vi "transmit messages.vi"(5 "extended ID?":bool, 6 "Network":T1(ring), 7 "Arb ID":u32, 8 "error in":errorcluster, 9 "Number of \nData Bytes":i32, 10 "hObject In":i32, 11 "Data":u8[](array[numeric])) -> (0 "error out":errorcluster, 3 "hObject Out":i32)   [LabVIEW 2018]
uses:
  ctl networkid.ctl
  ctl StatusBitfield.ctl
panel:
  out "*(type *) &x":i32[](array[numeric])
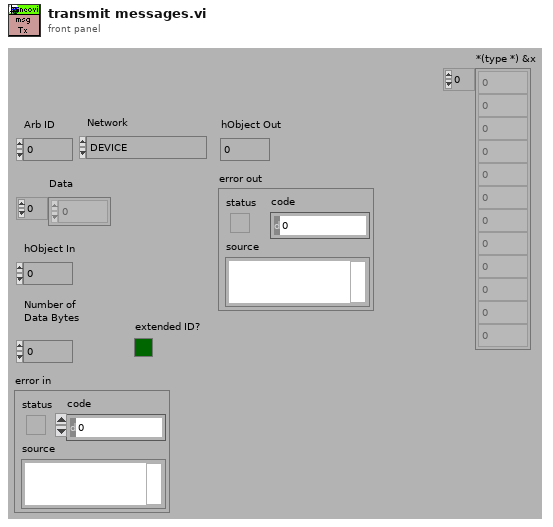
[diagram p1: front panel]
types:
  T1 = enum16{"DEVICE", "HSCAN", "MSCAN", "SWCAN", "LSFTCAN", "FORDSCP", "J1708", "JVPW", "ISO", "FIRE_HSCAN2", "FIRE_MSCAN1", "FIRE_HSCAN3", "FIRE_LIN2", "FIRE_LIN3", "FIRE_LIN4"}
  T2 = typedef "ctl NetworkID.ctl" = i8
  T3 = typedef "ctl StatusBitfield.ctl" = enum32{"GlobalError", "Tx", "XtdFrame", "RemoteFrame", "ErrCRCError", "CANErrorPassive", "ErrIncompleteFrame", "ErrLostArbitration", "Undefined", "CANBusOff", "CANErrorWarning", "BusShortedPlus", "BusShortedGnd", "CheckSumError", "ErrBadMessageBitTimeError", "IFRData", "HardwareCommError", "ExpectedLengthError", "IncomingNoMatch", "Break", "AVT_VSIRecOverflow", "TestTrigger", "AudioCommentType", "GPSDataValue", "AnalogDigitalInputValue", "TextCommentType", "NetworkMessageType", "VSI_TxUnderRun", "VSI_IFR_CRCBit", "StatusInitMessage", "HighSpeed"}
  T4 = typedef "ctl spymessage.ctl" = cluster{"StatusBitField":u32, "StatusBitField2":u32, "TimeHardware":u32, "TimeHardware2":u32, "TimeSystem":u32, "TimeSystem2":u32, "TimeStampHardwareID":u8, "TimeStampHardwareID2":u8, "NetworkID":u8, "NodeID":u8, "Protocol":u8, "MessagePieceID":u8, "ColorID":u8, "NumberBytesHeader":u8, "NumberBytesData":u8, "DescriptionID":u16, "ArbIDOrHeader":u32, "Data [8]":u8[], "AckBytes [8]":u8[], "Value":sgl, "MiscData":u8}
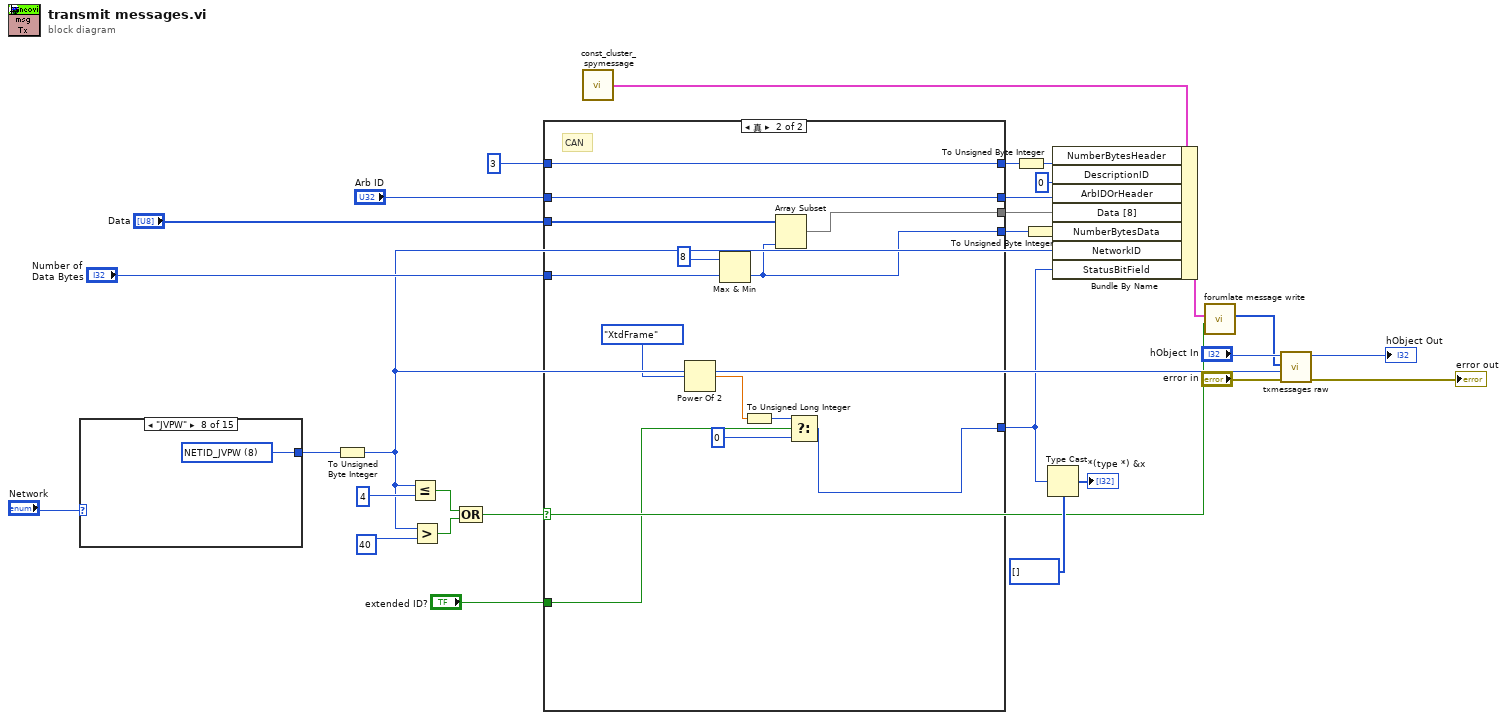
[diagram p0: block diagram]
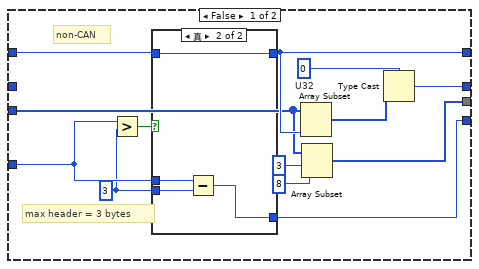
[diagram p2: hidden frame]
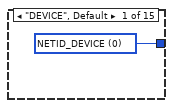
[diagram p4: hidden frame]
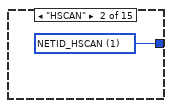
[diagram p5: hidden frame]
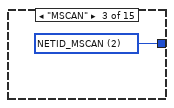
[diagram p6: hidden frame]
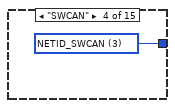
[diagram p7: hidden frame]
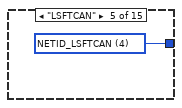
[diagram p8: hidden frame]
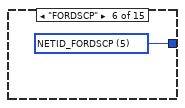
[diagram p9: hidden frame]
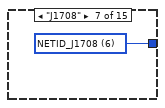
[diagram p10: hidden frame]
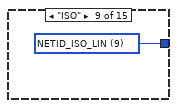
[diagram p11: hidden frame]
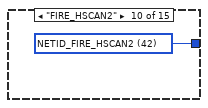
[diagram p12: hidden frame]
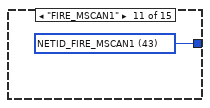
[diagram p13: hidden frame]
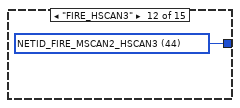
[diagram p14: hidden frame]
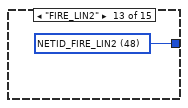
[diagram p15: hidden frame]
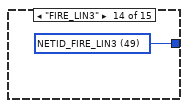
[diagram p16: hidden frame]
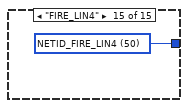
[diagram p17: hidden frame]
diagram:
  n1 = case shown="\"JVPW\"" "Network" {
    tunnel: [w31 w32 w33 w34 w35 w36 w37 w38 w39 w40 w41 w42 w43 w44 w45] -> w17
    frame "DEVICE", Default {
      w31 = T2 0 items=["NETID_DEVICE"=0, "NETID_HSCAN"=1, "NETID_MSCAN"=2, "NETID_SWCAN"=3, "NETID_LSFTCAN"=4, "NETID_FORDSCP"=5, "NETID_J1708"=6, "NETID_AUX"=7, "NETID_JVPW"=8, "NETID_ISO_LIN"=9, "NETID_ISOPIC"=10, "NETID_MAIN51"=11, "NETID_SCI"=13, "NETID_ISO2"=14, "NETID_FIRE_HSCAN1"=41, "NETID_FIRE_HSCAN2"=42, "NETID_FIRE_MSCAN1"=43, "NETID_FIRE_MSCAN2_HSCAN3"=44, "NETID_FIRE_SWCAN"=45, "NETID_FIRE_LSFT"=46, "NETID_FIRE_LIN1"=47, "NETID_FIRE_LIN2"=48, "NETID_FIRE_LIN3"=49, "NETID_FIRE_LIN4"=50] ("NetworID")
    }
    frame "HSCAN" {
      w32 = T2 1 items=["NETID_DEVICE"=0, "NETID_HSCAN"=1, "NETID_MSCAN"=2, "NETID_SWCAN"=3, "NETID_LSFTCAN"=4, "NETID_FORDSCP"=5, "NETID_J1708"=6, "NETID_AUX"=7, "NETID_JVPW"=8, "NETID_ISO_LIN"=9, "NETID_ISOPIC"=10, "NETID_MAIN51"=11, "NETID_SCI"=13, "NETID_ISO2"=14, "NETID_FIRE_HSCAN1"=41, "NETID_FIRE_HSCAN2"=42, "NETID_FIRE_MSCAN1"=43, "NETID_FIRE_MSCAN2_HSCAN3"=44, "NETID_FIRE_SWCAN"=45, "NETID_FIRE_LSFT"=46, "NETID_FIRE_LIN1"=47, "NETID_FIRE_LIN2"=48, "NETID_FIRE_LIN3"=49, "NETID_FIRE_LIN4"=50] ("NetworID")
    }
    frame "MSCAN" {
      w33 = T2 2 items=["NETID_DEVICE"=0, "NETID_HSCAN"=1, "NETID_MSCAN"=2, "NETID_SWCAN"=3, "NETID_LSFTCAN"=4, "NETID_FORDSCP"=5, "NETID_J1708"=6, "NETID_AUX"=7, "NETID_JVPW"=8, "NETID_ISO_LIN"=9, "NETID_ISOPIC"=10, "NETID_MAIN51"=11, "NETID_SCI"=13, "NETID_ISO2"=14, "NETID_FIRE_HSCAN1"=41, "NETID_FIRE_HSCAN2"=42, "NETID_FIRE_MSCAN1"=43, "NETID_FIRE_MSCAN2_HSCAN3"=44, "NETID_FIRE_SWCAN"=45, "NETID_FIRE_LSFT"=46, "NETID_FIRE_LIN1"=47, "NETID_FIRE_LIN2"=48, "NETID_FIRE_LIN3"=49, "NETID_FIRE_LIN4"=50] ("NetworID")
    }
    frame "SWCAN" {
      w34 = T2 3 items=["NETID_DEVICE"=0, "NETID_HSCAN"=1, "NETID_MSCAN"=2, "NETID_SWCAN"=3, "NETID_LSFTCAN"=4, "NETID_FORDSCP"=5, "NETID_J1708"=6, "NETID_AUX"=7, "NETID_JVPW"=8, "NETID_ISO_LIN"=9, "NETID_ISOPIC"=10, "NETID_MAIN51"=11, "NETID_SCI"=13, "NETID_ISO2"=14, "NETID_FIRE_HSCAN1"=41, "NETID_FIRE_HSCAN2"=42, "NETID_FIRE_MSCAN1"=43, "NETID_FIRE_MSCAN2_HSCAN3"=44, "NETID_FIRE_SWCAN"=45, "NETID_FIRE_LSFT"=46, "NETID_FIRE_LIN1"=47, "NETID_FIRE_LIN2"=48, "NETID_FIRE_LIN3"=49, "NETID_FIRE_LIN4"=50] ("NetworID")
    }
    frame "LSFTCAN" {
      w35 = T2 4 items=["NETID_DEVICE"=0, "NETID_HSCAN"=1, "NETID_MSCAN"=2, "NETID_SWCAN"=3, "NETID_LSFTCAN"=4, "NETID_FORDSCP"=5, "NETID_J1708"=6, "NETID_AUX"=7, "NETID_JVPW"=8, "NETID_ISO_LIN"=9, "NETID_ISOPIC"=10, "NETID_MAIN51"=11, "NETID_SCI"=13, "NETID_ISO2"=14, "NETID_FIRE_HSCAN1"=41, "NETID_FIRE_HSCAN2"=42, "NETID_FIRE_MSCAN1"=43, "NETID_FIRE_MSCAN2_HSCAN3"=44, "NETID_FIRE_SWCAN"=45, "NETID_FIRE_LSFT"=46, "NETID_FIRE_LIN1"=47, "NETID_FIRE_LIN2"=48, "NETID_FIRE_LIN3"=49, "NETID_FIRE_LIN4"=50] ("NetworID")
    }
    frame "FORDSCP" {
      w36 = T2 5 items=["NETID_DEVICE"=0, "NETID_HSCAN"=1, "NETID_MSCAN"=2, "NETID_SWCAN"=3, "NETID_LSFTCAN"=4, "NETID_FORDSCP"=5, "NETID_J1708"=6, "NETID_AUX"=7, "NETID_JVPW"=8, "NETID_ISO_LIN"=9, "NETID_ISOPIC"=10, "NETID_MAIN51"=11, "NETID_SCI"=13, "NETID_ISO2"=14, "NETID_FIRE_HSCAN1"=41, "NETID_FIRE_HSCAN2"=42, "NETID_FIRE_MSCAN1"=43, "NETID_FIRE_MSCAN2_HSCAN3"=44, "NETID_FIRE_SWCAN"=45, "NETID_FIRE_LSFT"=46, "NETID_FIRE_LIN1"=47, "NETID_FIRE_LIN2"=48, "NETID_FIRE_LIN3"=49, "NETID_FIRE_LIN4"=50] ("NetworID")
    }
    frame "J1708" {
      w37 = T2 6 items=["NETID_DEVICE"=0, "NETID_HSCAN"=1, "NETID_MSCAN"=2, "NETID_SWCAN"=3, "NETID_LSFTCAN"=4, "NETID_FORDSCP"=5, "NETID_J1708"=6, "NETID_AUX"=7, "NETID_JVPW"=8, "NETID_ISO_LIN"=9, "NETID_ISOPIC"=10, "NETID_MAIN51"=11, "NETID_SCI"=13, "NETID_ISO2"=14, "NETID_FIRE_HSCAN1"=41, "NETID_FIRE_HSCAN2"=42, "NETID_FIRE_MSCAN1"=43, "NETID_FIRE_MSCAN2_HSCAN3"=44, "NETID_FIRE_SWCAN"=45, "NETID_FIRE_LSFT"=46, "NETID_FIRE_LIN1"=47, "NETID_FIRE_LIN2"=48, "NETID_FIRE_LIN3"=49, "NETID_FIRE_LIN4"=50] ("NetworID")
    }
    frame "JVPW" {
      w38 = T2 8 items=["NETID_DEVICE"=0, "NETID_HSCAN"=1, "NETID_MSCAN"=2, "NETID_SWCAN"=3, "NETID_LSFTCAN"=4, "NETID_FORDSCP"=5, "NETID_J1708"=6, "NETID_AUX"=7, "NETID_JVPW"=8, "NETID_ISO_LIN"=9, "NETID_ISOPIC"=10, "NETID_MAIN51"=11, "NETID_SCI"=13, "NETID_ISO2"=14, "NETID_FIRE_HSCAN1"=41, "NETID_FIRE_HSCAN2"=42, "NETID_FIRE_MSCAN1"=43, "NETID_FIRE_MSCAN2_HSCAN3"=44, "NETID_FIRE_SWCAN"=45, "NETID_FIRE_LSFT"=46, "NETID_FIRE_LIN1"=47, "NETID_FIRE_LIN2"=48, "NETID_FIRE_LIN3"=49, "NETID_FIRE_LIN4"=50] ("NetworID")
    }
    frame "ISO" {
      w39 = T2 9 items=["NETID_DEVICE"=0, "NETID_HSCAN"=1, "NETID_MSCAN"=2, "NETID_SWCAN"=3, "NETID_LSFTCAN"=4, "NETID_FORDSCP"=5, "NETID_J1708"=6, "NETID_AUX"=7, "NETID_JVPW"=8, "NETID_ISO_LIN"=9, "NETID_ISOPIC"=10, "NETID_MAIN51"=11, "NETID_SCI"=13, "NETID_ISO2"=14, "NETID_FIRE_HSCAN1"=41, "NETID_FIRE_HSCAN2"=42, "NETID_FIRE_MSCAN1"=43, "NETID_FIRE_MSCAN2_HSCAN3"=44, "NETID_FIRE_SWCAN"=45, "NETID_FIRE_LSFT"=46, "NETID_FIRE_LIN1"=47, "NETID_FIRE_LIN2"=48, "NETID_FIRE_LIN3"=49, "NETID_FIRE_LIN4"=50] ("NetworID")
    }
    frame "FIRE_HSCAN2" {
      w40 = T2 42 items=["NETID_DEVICE"=0, "NETID_HSCAN"=1, "NETID_MSCAN"=2, "NETID_SWCAN"=3, "NETID_LSFTCAN"=4, "NETID_FORDSCP"=5, "NETID_J1708"=6, "NETID_AUX"=7, "NETID_JVPW"=8, "NETID_ISO_LIN"=9, "NETID_ISOPIC"=10, "NETID_MAIN51"=11, "NETID_SCI"=13, "NETID_ISO2"=14, "NETID_FIRE_HSCAN1"=41, "NETID_FIRE_HSCAN2"=42, "NETID_FIRE_MSCAN1"=43, "NETID_FIRE_MSCAN2_HSCAN3"=44, "NETID_FIRE_SWCAN"=45, "NETID_FIRE_LSFT"=46, "NETID_FIRE_LIN1"=47, "NETID_FIRE_LIN2"=48, "NETID_FIRE_LIN3"=49, "NETID_FIRE_LIN4"=50] ("NetworID")
    }
    frame "FIRE_MSCAN1" {
      w41 = T2 43 items=["NETID_DEVICE"=0, "NETID_HSCAN"=1, "NETID_MSCAN"=2, "NETID_SWCAN"=3, "NETID_LSFTCAN"=4, "NETID_FORDSCP"=5, "NETID_J1708"=6, "NETID_AUX"=7, "NETID_JVPW"=8, "NETID_ISO_LIN"=9, "NETID_ISOPIC"=10, "NETID_MAIN51"=11, "NETID_SCI"=13, "NETID_ISO2"=14, "NETID_FIRE_HSCAN1"=41, "NETID_FIRE_HSCAN2"=42, "NETID_FIRE_MSCAN1"=43, "NETID_FIRE_MSCAN2_HSCAN3"=44, "NETID_FIRE_SWCAN"=45, "NETID_FIRE_LSFT"=46, "NETID_FIRE_LIN1"=47, "NETID_FIRE_LIN2"=48, "NETID_FIRE_LIN3"=49, "NETID_FIRE_LIN4"=50] ("NetworID")
    }
    frame "FIRE_HSCAN3" {
      w42 = T2 44 items=["NETID_DEVICE"=0, "NETID_HSCAN"=1, "NETID_MSCAN"=2, "NETID_SWCAN"=3, "NETID_LSFTCAN"=4, "NETID_FORDSCP"=5, "NETID_J1708"=6, "NETID_AUX"=7, "NETID_JVPW"=8, "NETID_ISO_LIN"=9, "NETID_ISOPIC"=10, "NETID_MAIN51"=11, "NETID_SCI"=13, "NETID_ISO2"=14, "NETID_FIRE_HSCAN1"=41, "NETID_FIRE_HSCAN2"=42, "NETID_FIRE_MSCAN1"=43, "NETID_FIRE_MSCAN2_HSCAN3"=44, "NETID_FIRE_SWCAN"=45, "NETID_FIRE_LSFT"=46, "NETID_FIRE_LIN1"=47, "NETID_FIRE_LIN2"=48, "NETID_FIRE_LIN3"=49, "NETID_FIRE_LIN4"=50] ("NetworID")
    }
    frame "FIRE_LIN2" {
      w43 = T2 48 items=["NETID_DEVICE"=0, "NETID_HSCAN"=1, "NETID_MSCAN"=2, "NETID_SWCAN"=3, "NETID_LSFTCAN"=4, "NETID_FORDSCP"=5, "NETID_J1708"=6, "NETID_AUX"=7, "NETID_JVPW"=8, "NETID_ISO_LIN"=9, "NETID_ISOPIC"=10, "NETID_MAIN51"=11, "NETID_SCI"=13, "NETID_ISO2"=14, "NETID_FIRE_HSCAN1"=41, "NETID_FIRE_HSCAN2"=42, "NETID_FIRE_MSCAN1"=43, "NETID_FIRE_MSCAN2_HSCAN3"=44, "NETID_FIRE_SWCAN"=45, "NETID_FIRE_LSFT"=46, "NETID_FIRE_LIN1"=47, "NETID_FIRE_LIN2"=48, "NETID_FIRE_LIN3"=49, "NETID_FIRE_LIN4"=50] ("NetworID")
    }
    frame "FIRE_LIN3" {
      w44 = T2 49 items=["NETID_DEVICE"=0, "NETID_HSCAN"=1, "NETID_MSCAN"=2, "NETID_SWCAN"=3, "NETID_LSFTCAN"=4, "NETID_FORDSCP"=5, "NETID_J1708"=6, "NETID_AUX"=7, "NETID_JVPW"=8, "NETID_ISO_LIN"=9, "NETID_ISOPIC"=10, "NETID_MAIN51"=11, "NETID_SCI"=13, "NETID_ISO2"=14, "NETID_FIRE_HSCAN1"=41, "NETID_FIRE_HSCAN2"=42, "NETID_FIRE_MSCAN1"=43, "NETID_FIRE_MSCAN2_HSCAN3"=44, "NETID_FIRE_SWCAN"=45, "NETID_FIRE_LSFT"=46, "NETID_FIRE_LIN1"=47, "NETID_FIRE_LIN2"=48, "NETID_FIRE_LIN3"=49, "NETID_FIRE_LIN4"=50] ("NetworID")
    }
    frame "FIRE_LIN4" {
      w45 = T2 50 items=["NETID_DEVICE"=0, "NETID_HSCAN"=1, "NETID_MSCAN"=2, "NETID_SWCAN"=3, "NETID_LSFTCAN"=4, "NETID_FORDSCP"=5, "NETID_J1708"=6, "NETID_AUX"=7, "NETID_JVPW"=8, "NETID_ISO_LIN"=9, "NETID_ISOPIC"=10, "NETID_MAIN51"=11, "NETID_SCI"=13, "NETID_ISO2"=14, "NETID_FIRE_HSCAN1"=41, "NETID_FIRE_HSCAN2"=42, "NETID_FIRE_MSCAN1"=43, "NETID_FIRE_MSCAN2_HSCAN3"=44, "NETID_FIRE_SWCAN"=45, "NETID_FIRE_LSFT"=46, "NETID_FIRE_LIN1"=47, "NETID_FIRE_LIN2"=48, "NETID_FIRE_LIN3"=49, "NETID_FIRE_LIN4"=50] ("NetworID")
    }
  }
  n2 = To Unsigned Byte Integer(number=w17) -> (unsigned 8bit integer=w6:u8)
  n3 = Less Or Equal?(x=w6, y=u8 4) -> (x <= y?=w19:bool)
  n4 = Greater?(x=w6, y=u8 40) -> (0:w18:bool)
  n5 = Compound Arithmetic op=OR(w19, w18) -> (w1:bool)
  n6 = case shown="真" w1 {
    tunnel: "extended ID?" -> [_ w75]
    tunnel: [_ w64] -> w5
    tunnel: "Number of \nData Bytes" -> [w58 w74]
    tunnel: [w53 w70] -> w15
    tunnel: [w54 w72] -> w12
    tunnel: 3 ("NumberBytesHeader") -> [w55 w72]
    tunnel: [w52 w69] -> w10
    tunnel: "Data" -> [w49 w71]
    tunnel: "Arb ID" -> [_ w68]
    tunnel: [w47 w68] -> w7
    frame False {
      w48 = u32 0  # U32
      w57 = 3 ("y")
      # "max header = 3 bytes"
      # "non-CAN"
      n7 = Greater?(x=w58, y=w57) -> (0:w56:bool)
      n8 = case shown="真" w56 {
        tunnel: w58 -> [w59 w63]
        tunnel: w57 -> [_ w62]
        tunnel: [_ w61] -> w53
        tunnel: w55 -> [_ w60]
        tunnel: [w59 w60] -> w54
        frame False {
          # "only header data"
        }
        frame True {
          n9 = Subtract(x=w63, y=w62) -> (x-y=w61:i32)
        }
      }
      n10 = Array Subset(array=w49, length=w54) -> (w46:u8[])  [unwired: 1 in]
      n11 = Array Subset(array=w49, index=3, length=8) -> (w52:u8[])
      n12 = Type Cast(type=w48, x=w46) -> (*(type *) &x=w47:u32)
    }
    frame True {
      # "CAN"
      n13 = Power Of 2(x=ctl_StatusBitfield."XtdFrame" ("Enum")) -> (2^x=w66:dbl)
      n14 = Max & Min(x=8, y=w74) -> (min(x,y)=w70:i32)  [unwired: 1 out]
      n15 = To Unsigned Long Integer(number=w66) -> (unsigned 32bit integer=w65:u32)
      n16 = Array Subset(array=w71, length=w70) -> (w69:u8[])  [unwired: 1 in]
      n17 = Select(t=w65, s=w75, f=u32 0) -> (s? t:f=w64:u32)
    }
  }
  n18 = call "const_cluster_spymessage.vi"() -> ("SpyMessage{}"=w28:T4)
  n19 = To Unsigned Byte Integer(number=w12) -> (unsigned 8bit integer=w11:u8)
  n20 = To Unsigned Byte Integer(number=w15) -> (unsigned 8bit integer=w14:u8)
  n21 = Type Cast(type=i32[] [], x=w5) -> (*(type *) &x=→"*(type *) &x":i32[])
  n22 = Bundle By Name(cluster=w28, "NumberBytesHeader"=w11, "DescriptionID"=u16 0, "ArbIDOrHeader"=w7, "Data [8]"=w10, "NumberBytesData"=w14, "NetworkID"=w6, "StatusBitField"=w5) -> (w23:T4)
  n23 = call "forumlate message write.vi"("can?"=w1, "SpyMessage{}"=w23) -> ("Messages Raw OUT"=w22:u8[])  [unwired: 9 out]
  n24 = call "txmessages raw.vi"("error in (no error)"="error in", "networkID"=w6, "Messages Raw In"=w22, "hObject"="hObject In") -> ("error out"=→"error out":errorcluster, "hObject Out"=→"hObject Out":i32)  [unwired: 6 out]
